vi "File_ToXML.vi"(8 "error in (no error)":errorcluster, 11 "File in":refnum<class "File.lvclass">) -> (0 "error out":errorcluster, 2 "XML String":string, 3 "File out":refnum<class "File.lvclass">)   [LabVIEW 2023, in "File.lvclass"]
doc: "Export the current file definition to XML."
uses:
  File.lvclass
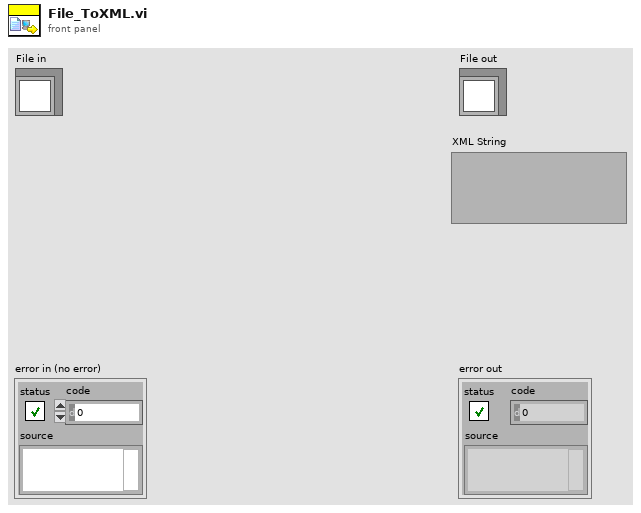
[diagram p1: front panel]
types:
  T1 = typedef "FileAsCluster.ctl" = cluster{"Name":string, "Directory":string, "Date Captured":string, "Groups":T2[], "Meta Data":T5[], "File Start Time":timestamp, "appended path":path}
  T2 = typedef "GroupAsCluster.ctl" = cluster{"Name":string, "Channels":T3[], "Meta Data":T5[]}
  T3 = typedef "ChannelAsCluster.ctl" = cluster{"Name":string, "Data Reference":T4, "Wfm?":bool, "Decimation":i32, "Current Value":dbl, "Meta Data":T5[], "WfmPath":string}
  T4 = typedef "Custom Device API.lvlib/Data Reference.ctl" = i32
  T5 = typedef "Meta Data.ctl" = cluster{"Key":string, "Value":string}
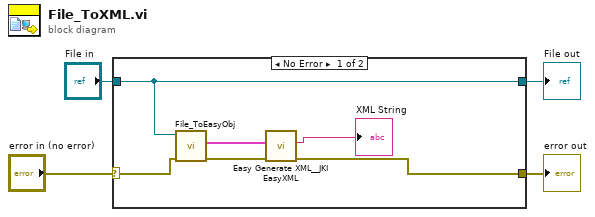
[diagram p0: block diagram]
diagram:
  n1 = case shown="No Error" "error in (no error)" {
    selector: "error in (no error)" -> [w6 w12]
    tunnel: [w9 w12] -> w3
    tunnel: [w5 w11] -> w1
    tunnel: "File in" -> [w5 w11]
    frame No Error {
      n2 = call-dynamic "File_ToEasyObj.vi"("error in (no error)"=w6, "File in"=w5) -> ("error out"=w7:errorcluster, "output cluster"=w8:T1)  [unwired: 7 in, 1 out]
      n3 = call <vilib>:"Easy Generate XML__JKI EasyXML.vi"("error in (no error)"=w7, "LabVIEW Data"=w8) -> ("error out"=w9:errorcluster, "XML String"=→"XML String":string)  [unwired: 8 in]
    }
    frame Error {
    }
  }
  "error out" <- w3
  "File out" <- w1
